vi "TDS读取波形.VI"() -> ()   [LabVIEW 2017]
uses:
  <vilib>/measure/matone.llb/Extract Single Tone Information 1 Chan.vi
  <vilib>/measure/NI_MAPro.lvlib
panel:
  out "幅值":dbl format="%.2p"
  in  "串口参数设置":enum32{"常用设置", "不常用的"}(tab)
  in  "VISA resource name":refnum<visa-resource-name>="COM1" caption="端口号"
  in  "baud rate":u32=9600 caption="波特率"
  in  "parity":u16(ring) caption="奇偶校验" items=["None", "Odd", "Even", "Mark", "Space"]
  in  "stop bits":u16(ring)=10 caption="停止位" items=["1.0"=10, "1.5"=15, "2.0"=20]
  in  "data bits":u16=8 caption="数据位" min=5 max=8 step=1
  in  "Input buffer size":u32=4096 caption="输入缓冲区大小"
  in  "要读的\n字节数":u32=1000 caption="所读字节数"
  in  "XOFF Character":u8=19 format="%.0x"
  in  "XON Character":u8=17 format="%.0x"
  in  "timeout (ms)":u32=10000
  in  "flow control":u16(ring) caption="流量控制" items=["None"=0, "XON/XOFF"=1, "RTS/CTS"=2, "DTR/DSR"=4]
  in  "termination char\n(0xA = '\\n' = LF)":u8=10 caption="EOL字串-LF" format="%.0x"
  out "YZEro":dbl
  out "单位":string
  out "YMUlt":dbl
  out "YOFf":dbl
  out "XZEro":dbl
  out "单位":string
  out "坐标偏移量":dbl
  out "DeltX":dbl
  out "示波器刻度":dbl
  out "频率":dbl caption="波形频率" format="%.2p"
  out "波形图":waveform(dbl)(graph)
  # "读取示波器当前坐标轴信息"
  # "X轴"
  # "Y轴"
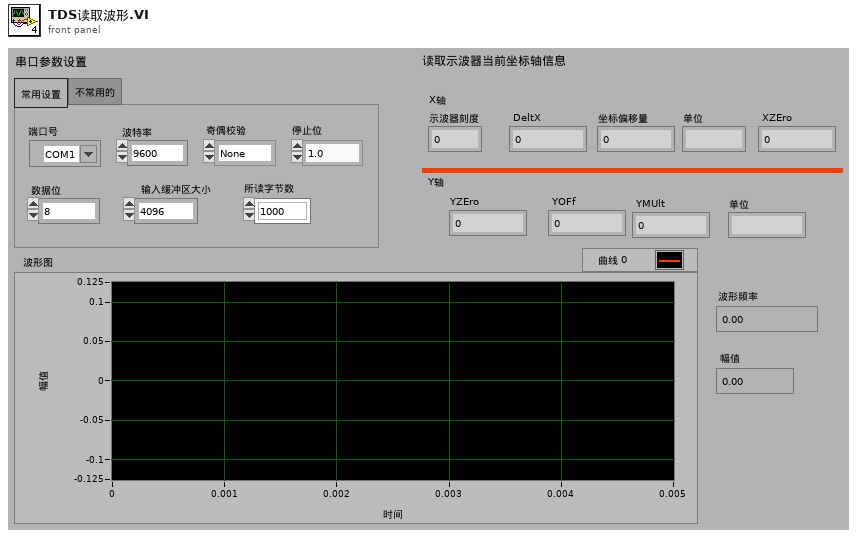
[diagram p1: front panel]
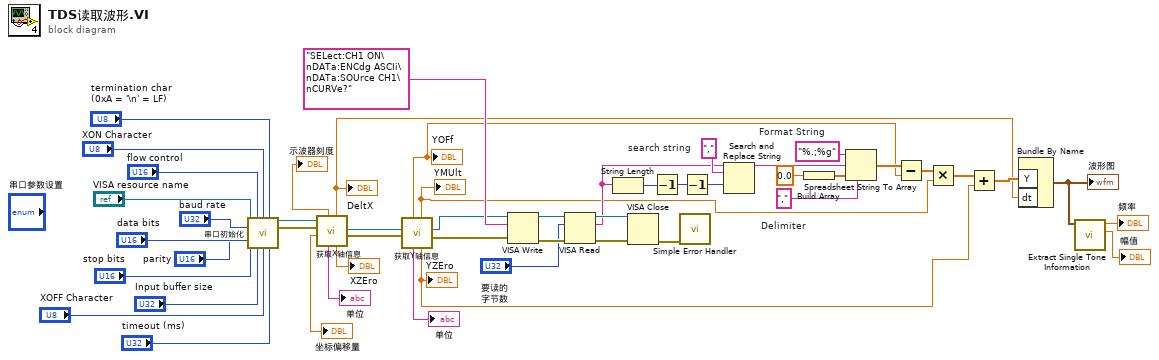
[diagram p0: block diagram]
diagram:
  w29 = ","  # search string
  w24 = ","  # Delimiter
  w32 = "%.;%g"  # Format String
  n1 = call "串口初始化.vi"("VISA resource name"="VISA resource name", "flow control"="flow control", "XON Character"="XON Character", "termination char\n(0xA = '\\n' = LF)"="termination char\n(0xA = '\\n' = LF)", "baud rate"="baud rate", "data bits"="data bits", "parity"="parity", "stop bits"="stop bits", "Input buffer size"="Input buffer size", "XOFF Character"="XOFF Character", "timeout (ms)"="timeout (ms)") -> ("VISA resource name out"=w18:refnum<visa-resource-name>, "错误输出"=w17:errorcluster)  [unwired: 3 in]
  n2 = call "获取X轴信息.vi"("错误输入（无错误）"=w17, "VISA资源名称"=w18) -> ("错误输出"=w15:errorcluster, "VISA资源名称输出"=w16:refnum<visa-resource-name>, "XZEro"=→"XZEro":dbl, "DeltX"=w5:dbl, "XUNit"=→"单位":string, "示波器刻度"=→"示波器刻度":dbl, "坐标偏移量"=→"坐标偏移量":dbl)  [unwired: 3 in]
  "DeltX" <- w5
  n3 = call "获取Y轴信息.vi"("错误输入（无错误）"=w15, "VISA资源名称"=w16) -> ("错误输出"=w13:errorcluster, "VISA资源名称输出"=w14:refnum<visa-resource-name>, "YZEro"=w2:dbl, "YMUlt"=w3:dbl, "YUNit"=→"单位":string, "YOFf"=w4:dbl)  [unwired: 4 in]
  "YOFf" <- w4
  "YMUlt" <- w3
  "YZEro" <- w2
  n4 = VISA Write(VISA resource name=w14, write buffer="SELect:CH1 ON\nDATa:ENCdg ASCIi\nDATa:SOUrce CH1\nCURVe?" ("string to write"), error in (no error)=w13) -> (VISA resource name out=w38:refnum<visa-resource-name>, error out=w37:errorcluster)  [unwired: 1 out]
  n5 = VISA Read(VISA resource name=w38, byte count="要读的\n字节数", error in (no error)=w37) -> (VISA resource name out=w36:refnum<visa-resource-name>, read buffer=w23:string, error out=w35:errorcluster)  [unwired: 1 out]
  n6 = String Length(string=w23) -> (length=w25:i32)
  n7 = VISA Close(VISA resource name=w36, error in (no error)=w35) -> (error out=w39:errorcluster)
  n8 = Decrement(x=w25) -> (x-1=w26:i32)
  n9 = call <vilib>:"Simple Error Handler.vi"("error in (no error)"=w39) -> ()  [unwired: 4 in, 5 out]
  n10 = Decrement(x=w26) -> (x-1=w27:i32)
  n11 = Search and Replace String(input string=w23, search string=w29, offset=w27) -> (result string=w28:string)  [unwired: 5 in, 3 out]
  n12 = Build Array(0.0) -> (w30:dbl[])
  n13 = Spreadsheet String To Array(delimiter (Tab)=w24, format string=w32, spreadsheet string=w28, array type (2D Dbl)=w30) -> (array=w22:dbl[])
  n14 = Subtract(x=w22, y=w4) -> (x-y=w21:dbl[])
  n15 = Multiply(x=w21, y=w3) -> (x*y=w6:dbl[])
  n16 = Add(x=w6, y=w2) -> (x+y=w7:dbl[])
  n17 = Bundle By Name("Y"=w7, "dt"=w5) -> (w20:waveform(dbl))  [unwired: 1 in]
  "波形图" <- w20
  n18 = call-poly <vilib>:"Extract Single Tone Information.vi"("time signal in"=w20) -> ("detected amplitude"=→"幅值":dbl, "detected frequency"=→"频率":dbl)  [unwired: 5 in, 4 out]
